vi "Create.vi"(7 "Direction":T1, 8 "error in (no error)":errorcluster, 9 "Custom Config Data":u8[](array[numeric]), 10 "Name":string, 11 "CIF_Fifo_U8 in":refnum<class "CIF_Fifo_CAN_Multi.lvclass">) -> (0 "error out":errorcluster, 3 "CIF_Fifo_U8 out":refnum<class "CIF_Fifo_CAN_Multi.lvclass">)   [LabVIEW 2021, in "CIF_Fifo_CAN_Multi.lvclass"]
uses:
  CIF_Fifo_CAN_Multi.lvclass
  D:/dev/Packages/Channel_Manager/src/CIFChannels/CIFChannels.lvclass
  D:/dev/Packages/Channel_Manager/src/CIF_NIChn/NIChn/CIF_NIChn.lvclass
  D:/dev/Packages/Channel_Manager/src/CIF_NIChn/FIFO_U8/CIF_NIChn_Fifo_U8.lvclass
  CIFChannels/Typedef/Direction.ctl
  CIFChannels/Typedef/Disconnect Behavior.ctl
  CIFChannels/CIFChannels.lvclass/CIFChannels.ctl
  <vilib>/CIF Foundation/CIF Utilities/Statistics/I64/Stats_I64_CIF_U.lvclass/Stats_I64_CIF_U.ctl
  CIFChannels/Typedef/Channel State.ctl
  NIChn/CIF_NIChn.lvclass/CIF_NIChn.ctl
  FIFO_U8/CIF_NIChn_Fifo_U8.lvclass/CIF_NIChn_Fifo_U8.ctl
  6cf79c70-debc-41de-b122-58e2a501a1fe.vi
  CIFChannels/Accessors/Write Channel State.vi
  NIChn/Accessors/Write CIF Channel.vi
  CIFChannels/Accessors/Write Channel Benchmark.vi
  CIFChannels/Accessors/Write Flatten Benchmark.vi
  FIFO_U8/Accessors/Write Payload.vi
  CIFChannels/Accessors/Write Type.vi
  ChannelCommon/Utilities/Unflatten FIFO Config.vi
  CIFChannels/Utilities/Apply Flags.vi
  CIFChannels/Accessors/Write Channel Class.vi
  CIFChannels/Accessors/Write Direction.vi
  CIFChannels/Accessors/Write Tag Disconnect Behavior.vi
  CIFChannels/Accessors/Write Name.vi
  CIFChannels/Accessors/Write Custom Config Data.vi
  <vilib>/CIF Foundation/CIF Channels/CIFChannels/SubVIs/Add Error.vi
  6cf79c70-debc-41de-b122-58e2a501a1fe.vi/c28b0ead-42ad-4072-80a2-aca7f2bd7ce3.vi
  <vilib>/CIF Foundation/CIF Channels/CIFChannels/SubVIs/CIFServices Fill In Error Info Ex.vi
  <vilib>/CIF Foundation/CIF Channels/CIFChannels/SubVIs/Get dll Path.vi
  <vilib>/CIF Foundation/CIF Utilities/DataTypes/Unflatten U64.vi
  ChannelCommon/Utilities/Expand FIFO Flags.vi
  <vilib>/CIF Foundation/CIF Utilities/Errors/Append Error Location.vi
  <vilib>/CIF Foundation/CIF Utilities/Statistics/I64/Stats_I64_CIF_U.lvclass
  CIF_Fifo_CAN_Multi.lvclass/CIF_Fifo_CAN_Multi.ctl
  CIFChannels/CIFChannels.lvclass
  ChannelCommon/ChannelCommon.lvlib
  FIFO_CAN/CIF_NIChn_FifoCAN.lvclass
  D:/dev/Packages/Channel_Manager/src/CIF_NIChn/FIFO_CAN/CIF_NIChn_FifoCAN.lvclass
  D:/dev/Packages/Channel_Manager/src/CIF_NIChn/FIFO_CAN_Multi/CIF_Fifo_CAN_Multi.lvclass
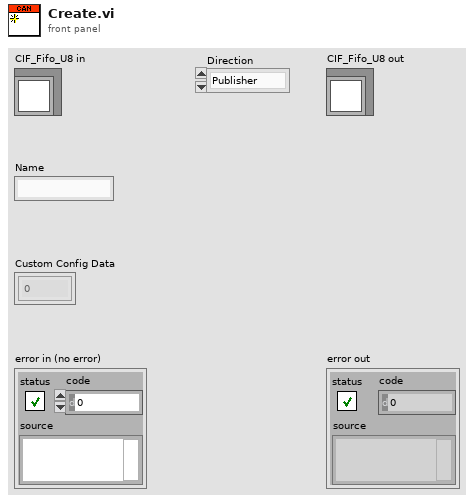
[diagram p1: front panel]
types:
  T1 = typedef "CIFChannels.lvclass/Direction.ctl" = enum16{"Publisher", "Subscriber"}
  T2 = typedef "CIFChannels.lvclass/Disconnect Behavior.ctl" = enum16{"Default value", "Last value", "Error with default"}
  T3 = typedef "CIFChannels.lvclass/Channel State.ctl" = enum16{"Creating", "Disconnected", "Connecting", "Connected", "Destroyed"}
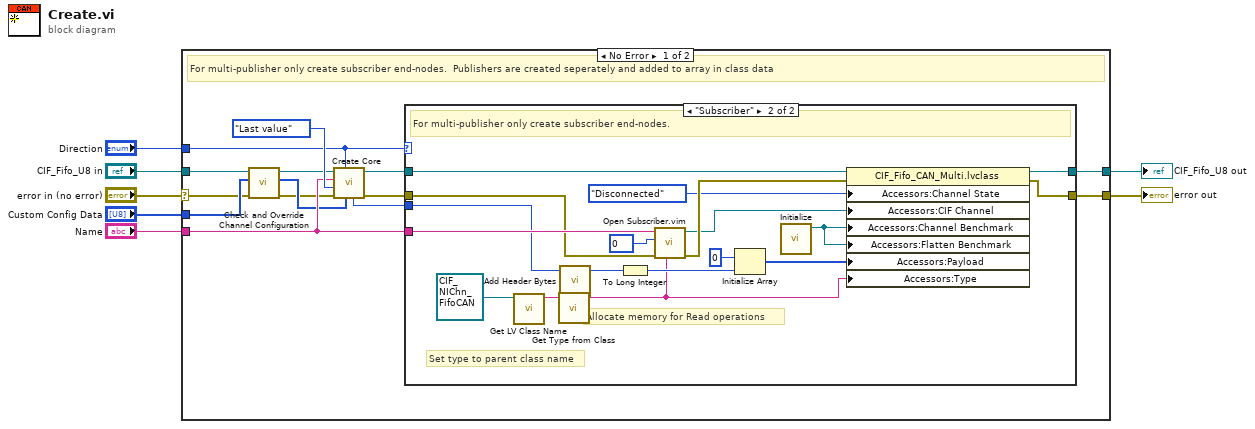
[diagram p0: block diagram]
diagram:
  n1 = case shown="No Error" "error in (no error)" {
    selector: "error in (no error)" -> [w15 w43]
    tunnel: [w9 w43] -> w2
    tunnel: [w10 w42] -> w1
    tunnel: "CIF_Fifo_U8 in" -> [w18 w42]
    tunnel: "Name" -> [w20 _]
    tunnel: "Direction" -> [w12 _]
    tunnel: "Custom Config Data" -> [w17 _]
    frame No Error {
      # "For multi-publisher only create subscriber end-nodes.  Publishers are created seperately and added to array in class data"
      n2 = call-dynamic "Check and Override Channel Configuration.vi"("error in (no error)"=w15, "Custom Config Data in"=w17, "CIF_NIChn_FifoCAN in"=w18) -> ("error out"=w14:errorcluster, "Custom Config Data out"=w16:u8[], "CIF_NIChn_FifoCAN out"=w13:refnum<class "CIF_Fifo_CAN_Multi.lvclass">)  [unwired: 6 in]
      n3 = call "Create Core.vi"("Custom Config Data"=w16, "Direction"=w12, "error in (no error)"=w14, "Disconnect Behavior"=Disconnect_Behavior."Last value", "Name"=w20, "CIFChannels in"=w13) -> ("error out"=w19:errorcluster, "CIFChannels out"=w11:refnum<class "CIF_Fifo_CAN_Multi.lvclass">, "Bytes/Msg"=w8:u64)  [unwired: 1 in, 2 out]
      n4 = case shown="\"Subscriber\"" w12 {
        tunnel: w20 -> [_ w41]
        tunnel: w19 -> [w23 w40]
        tunnel: w11 -> [w22 w35]
        tunnel: [w22 w30] -> w10
        tunnel: [w23 w29] -> w9
        tunnel: w8 -> [_ w25]
        frame "Publisher", Default {
          # "Publishers are created seperately and added to array in class data"
        }
        frame "Subscriber" {
          # "Set type to parent class name"
          # "Allocate memory for Read operations"
          # "For multi-publisher only create subscriber end-nodes."
          n5 = call <vilib>:"Get LV Class Name.vi"("object"=refnum<class "CIF_NIChn_FifoCAN.lvclass"> refnum ("CIF_NIChn_FIFO_DAQ in")) -> ("class name"=w28:string)  [unwired: 9 in, 1 out]
          n6 = call "Get Type from Class.vi"("Class"=w28) -> ("Channel Type"=w26:string)  [unwired: 4 in]
          n7 = call "Add Header Bytes.vi"("Bytes/Msg"=w25) -> ("Bytes/Msg with header"=w24:u64)  [unwired: 3 in]
          n8 = To Long Integer(number=w24) -> (32bit integer=w39:i32)
          n9 = call "Open Subscriber.vim"("Channel Type Description"=w26, "error in"=w40, "Input Type"=u8 0, "Channel Name"=w41) -> ("error out"=w34:errorcluster, "CIF Channel"=w32:refnum<k21>)  [unwired: 6 in]
          n10 = Initialize Array(u8 0 ("Numeric"), w39) -> (w31:u8[])
          n11 = call <vilib>:"Initialize.vi"() -> ("Stats_I64_CIF_U out"=w36:refnum<class "Stats_I64_CIF_U.lvclass">)  [unwired: 10 in, 1 out]
          n12 = property class="CIF_Fifo_CAN_Multi.lvclass"(reference=w35, error in=w34, "Accessors:Channel State"=Channel_State."Disconnected" ("Channel State"), "Accessors:CIF Channel"=w32, "Accessors:Channel Benchmark"=w36, "Accessors:Flatten Benchmark"=w36, "Accessors:Payload"=w31, "Accessors:Type"=w26) -> (reference out=w30:refnum<class "CIF_Fifo_CAN_Multi.lvclass">, error out=w29:errorcluster)
        }
      }
    }
    frame Error {
    }
  }
  "error out" <- w2
  "CIF_Fifo_U8 out" <- w1
